vi "Create Unique Module Identifier.vi"(11 "existing module identifiers":string[](array[string])) -> (3 "unique module identifier":string)   [LabVIEW 2020, in "Routing and Faulting Scripting.lvlib"]
uses:
  Routing and Faulting Scripting.lvlib
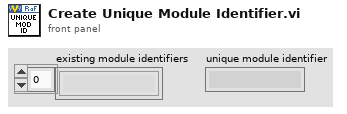
[diagram p1: front panel]
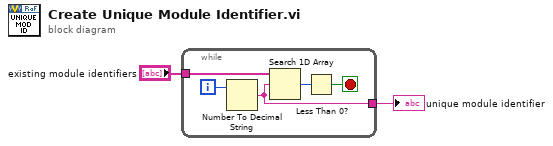
[diagram p0: block diagram]
diagram:
  n1 = while {
    tunnel: "existing module identifiers" -> [w6]
    tunnel: [w3] -> w2
    i -> [w7]
    stop <- w4 stop-if-true
    n2 = Number To Decimal String(number=w7) -> (decimal integer string=w3:string)  [unwired: 1 in]
    n3 = Search 1D Array(1D array=w6, element=w3) -> (index of element=w5:i32)  [unwired: 1 in]
    n4 = Less Than 0?(x=w5) -> (x < 0?=w4:bool)
  }
  "unique module identifier" <- w2
